vi "Calculate X Y Step Size.vi"(6 "Overlap Options":T3 {"Percent Overlap" max=50}, 7 "Scan Pattern":T1(ring), 8 "Error In":errorcluster, 10 "Y Axis":T2, 11 "X Axis":T2) -> (0 "Error Out":errorcluster, 1 "Array":cluster{"X":dbl, "Y":dbl}[](array[cluster]), 2 "Y Axis Out":T2, 3 "X Axis Out":T2)   [LabVIEW 2018]
panel:
  out "XY Graph":cluster{"X":dbl, "Y":dbl}[](graph)
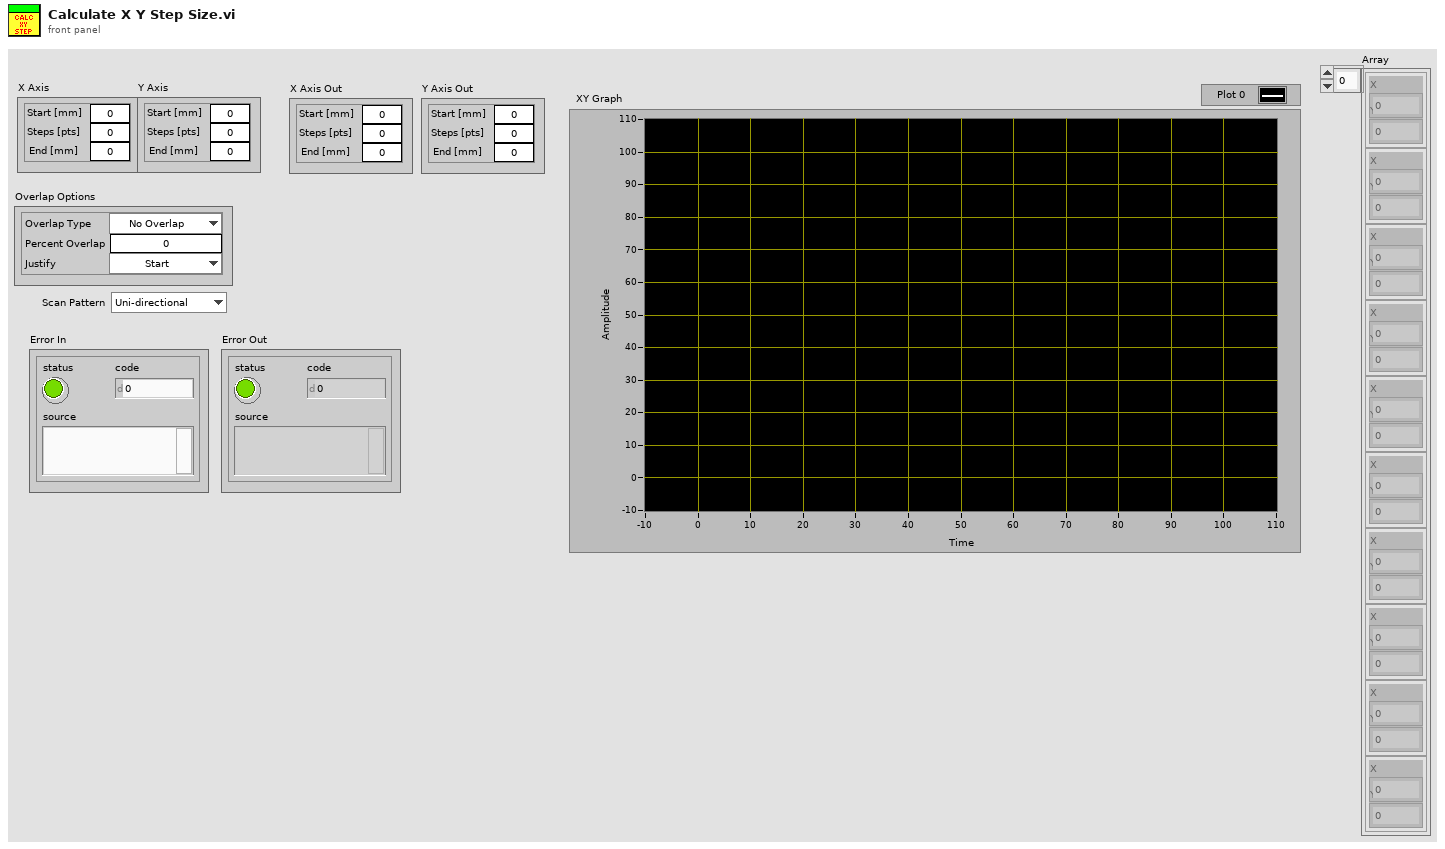
[diagram p1: front panel]
types:
  T1 = enum16{"Uni-directional", "Bi-Directional", "Spiral Out", "Spiral In"}
  T2 = cluster{"Start [mm]":dbl, "Steps [pts]":u16, "End [mm]":dbl}
  T3 = cluster{"Overlap Type":enum16{"No Overlap", "X Only", "Y Only", "X and Y"}, "Percent Overlap":u8, "Justify":enum16{"Start", "Center", "End"}}
  T4 = enum16{"No Overlap", "X Only", "Y Only", "X and Y"}
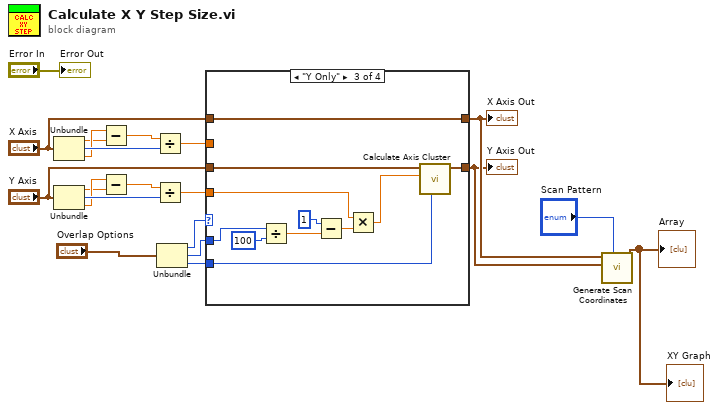
[diagram p0: block diagram]
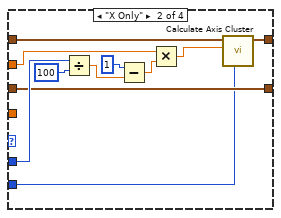
[diagram p3: hidden frame]
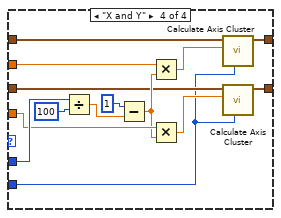
[diagram p4: hidden frame]
diagram:
  n1 = Unbundle("X Axis") -> ("Start [mm]"=w11:dbl, "Steps [pts]"=w19:u16, "End [mm]"=w12:dbl)
  n2 = Unbundle("Y Axis") -> ("Start [mm]"=w9:dbl, "Steps [pts]"=w17:u16, "End [mm]"=w10:dbl)
  n3 = Subtract(x=w12, y=w11) -> (x-y=w20:dbl)
  n4 = Subtract(x=w10, y=w9) -> (x-y=w18:dbl)
  n5 = Divide(x=w20, y=w19) -> (x/y=w13:dbl)
  n6 = Divide(x=w18, y=w17) -> (x/y=w14:dbl)
  n7 = Unbundle("Overlap Options") -> ("Overlap Type"=w16:T4, "Percent Overlap"=w15:u8, "Justify"=w5:enum16{"Start", "Center", "End"})
  n8 = case shown="\"Y Only\"" w16 {
    tunnel: w15 -> [_ w34 w45 w59]
    tunnel: w14 -> [_ _ w40 w55]
    tunnel: w13 -> [_ w30 _ w53]
    tunnel: "X Axis" -> [w23 w27 w39 w52]
    tunnel: "Y Axis" -> [w22 w28 w37 w51]
    tunnel: [w23 w25 w39 w48] -> w4
    tunnel: [w22 w28 w38 w47] -> w3
    tunnel: w5 -> [_ w24 w35 w46]
    frame "No Overlap", Default {
    }
    frame "X Only" {
      n9 = Divide(x=w34, y=u8 100) -> (x/y=w32:dbl)
      n10 = Subtract(x=u8 1 ("y"), y=w32) -> (x-y=w29:dbl)
      n11 = Multiply(x=w30, y=w29) -> (x*y=w26:dbl)
      n12 = call "Calculate Axis Cluster.vi"("Justify"=w24, "Step Size"=w26, "X Axis in"=w27) -> ("X Axis out"=w25:T2)  [unwired: 8 in]
    }
    frame "Y Only" {
      n13 = Divide(x=w45, y=u8 100) -> (x/y=w43:dbl)
      n14 = Subtract(x=u8 1 ("y"), y=w43) -> (x-y=w41:dbl)
      n15 = Multiply(x=w40, y=w41) -> (x*y=w36:dbl)
      n16 = call "Calculate Axis Cluster.vi"("Justify"=w35, "Step Size"=w36, "X Axis in"=w37) -> ("X Axis out"=w38:T2)  [unwired: 8 in]
    }
    frame "X and Y" {
      n17 = Divide(x=w59, y=u8 100) -> (x/y=w57:dbl)
      n18 = Subtract(x=u8 1 ("y"), y=w57) -> (x-y=w54:dbl)
      n19 = Multiply(x=w53, y=w54) -> (x*y=w50:dbl)
      n20 = Multiply(x=w55, y=w54) -> (x*y=w49:dbl)
      n21 = call "Calculate Axis Cluster.vi"("Justify"=w46, "Step Size"=w50, "X Axis in"=w52) -> ("X Axis out"=w48:T2)  [unwired: 8 in]
      n22 = call "Calculate Axis Cluster.vi"("Justify"=w46, "Step Size"=w49, "X Axis in"=w51) -> ("X Axis out"=w47:T2)  [unwired: 8 in]
    }
  }
  "X Axis Out" <- w4
  "Y Axis Out" <- w3
  n23 = call "Generate Scan Coordinates.vi"("Scan Pattern"="Scan Pattern", "Y Axis"=w3, "X Axis"=w4) -> ("Array"=→"XY Graph" →"Array":cluster{"X":dbl, "Y":dbl}[])  [unwired: 6 in, 2 out]
  "Error Out" <- "Error In"
